vi "Priority.vi"(8 "error in (no error)":errorcluster, 11 "Error Logger in":refnum<class "Error Logger.lvclass">) -> (0 "error out":errorcluster, 2 "Priority":u16, 3 "Error Logger out":refnum<class "Error Logger.lvclass">)   [LabVIEW 2020, in "Summer of LabVIEW.lvlib" / "Error Logger.lvclass"]
uses:
  Error Logger.lvclass
  Error Logger.lvclass/Error Logger.ctl
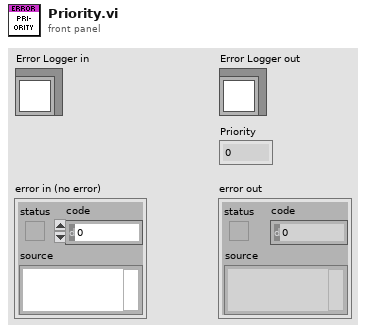
[diagram p1: front panel]
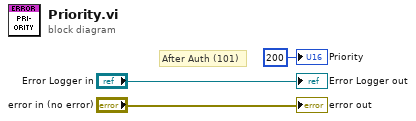
[diagram p0: block diagram]
diagram:
  # "After Auth (101)"
  "error out" <- "error in (no error)"
  "Error Logger out" <- "Error Logger in"
  "Priority" <- u16 200 ("Priority")
